vi "DCA Convert 1.5 to 1.8.vi"(1 "DCA 1.5 Test Parameters":T2={"Tag"="", "Use Instrument"=FALSE, "Quick Mode"=FALSE, "Topology"=enum."Pi", "Zo"=50.0, "Range"=0, "Resolution"=0, "Blank Screen"=FALSE, "Limits"=[], "Reports"={"Reports to Generate"=[], "Print Reports"=TRUE}, "Lock Topology"=FALSE, "Normalize"=TRUE, "ATTN Calc"=enum."Power"} {"Resolution" items=["Auto", "4 1/2", "5 1/2", "6 1/2"]; "Range" items=["Auto", "Min", "Max", "100", "1,000", "10,000", "100,000", "1,000,000", "10,000,000", "100,000,000"]}) -> (0 "DCA 1.8 Test Parameters":T1={"Tag"="", "Use Instrument"=FALSE, "Quick Mode"=FALSE, "Topology"=enum."Pi", "Zo"=50.0, "Range"=0, "Resolution"=0, "Blank Screen"=FALSE, "Limits"=[], "Datasheets"={"Datasheets to Generate"=[], "Print Datasheets"=TRUE}, "Lock Topology"=FALSE, "Normalize"=TRUE, "ATTN Calc"=enum."Power"} {"Resolution" items=["Auto", "4 1/2", "5 1/2", "6 1/2"]; "Range" items=["Auto", "Min", "Max", "100", "1,000", "10,000", "100,000", "1,000,000", "10,000,000", "100,000,000"]; "Limits"."Run" min=1 step=1})   [LabVIEW 2011]
uses:
  TypeDefs/DCA Test Parameters v1.5.ctl
  TypeDefs/DCA Test Parameters v1.8.ctl
panel:
  # "="
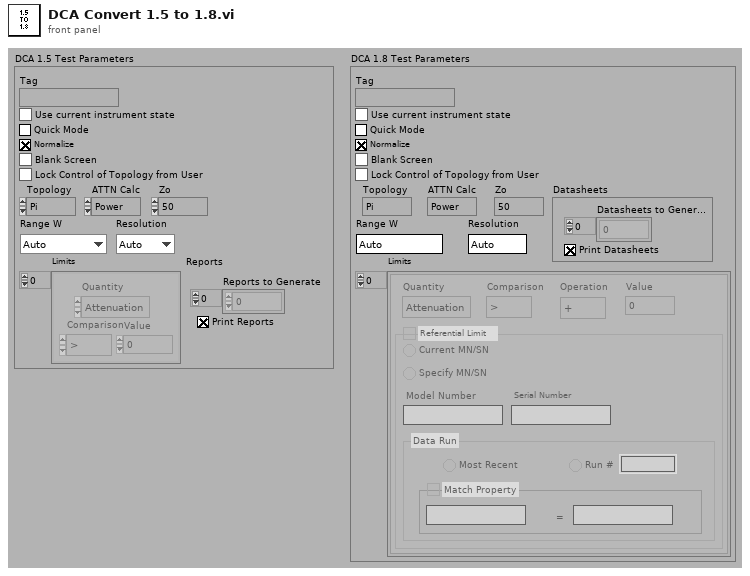
[diagram p1: front panel]
types:
  T1 = typedef "DCA Test Parameters v1.8.ctl" = cluster{"Tag":string, "Use Instrument":bool, "Quick Mode":bool, "Topology":enum32{"Pi", "T"}, "Zo":dbl, "Range":u16, "Resolution":u16, "Blank Screen":bool, "Limits":cluster{"Quantity":enum16{"Attenuation", "Zin", "Zout", "R1", "R2", "R3", "Rab", "Rac", "Rbc"}, "Comparison":enum16{">", ">=", "<", "<=", "+", "-"}, "Operation":enum16{"+", "-"}, "Value":dbl, "Ref Limit":bool, "Ref Type":enum32{"Current", "Specify"}, "Model":string, "Serial":string, "Run Type":enum32{"Most Recent", "Run #"}, "Run":i32, "Match Property":bool, "Property":string, "Property Value":string}[], "Datasheets":cluster{"Datasheets to Generate":i32[], "Print Datasheets":bool}, "Lock Topology":bool, "Normalize":bool, "ATTN Calc":enum32{"Power", "Voltage"}}
  T2 = typedef "DCA Test Parameters v1.5.ctl" = cluster{"Tag":string, "Use Instrument":bool, "Quick Mode":bool, "Topology":enum32{"Pi", "T"}, "Zo":dbl, "Range":u16, "Resolution":u16, "Blank Screen":bool, "Limits":cluster{"Quantity":enum16{"Attenuation", "Zin", "Zout", "R1", "R2", "R3", "Rab", "Rac", "Rbc"}, "Comparison":enum16{">", ">=", "<", "<=", "+", "-"}, "Value":dbl}[], "Reports":cluster{"Reports to Generate":i32[], "Print Reports":bool}, "Lock Topology":bool, "Normalize":bool, "ATTN Calc":enum32{"Power", "Voltage"}}
  T3 = cluster{"Quantity":enum16{"Attenuation", "Zin", "Zout", "R1", "R2", "R3", "Rab", "Rac", "Rbc"}, "Comparison":enum16{">", ">=", "<", "<=", "+", "-"}, "Operation":enum16{"+", "-"}, "Value":dbl, "Ref Limit":bool, "Ref Type":enum32{"Current", "Specify"}, "Model":string, "Serial":string, "Run Type":enum32{"Most Recent", "Run #"}, "Run":i32, "Match Property":bool, "Property":string, "Property Value":string}[]
  T4 = cluster{"Reports to Generate":i32[], "Print Reports":bool}
  T5 = cluster{"Quantity":enum16{"Attenuation", "Zin", "Zout", "R1", "R2", "R3", "Rab", "Rac", "Rbc"}, "Comparison":enum16{">", ">=", "<", "<=", "+", "-"}, "Value":dbl}[]
  T6 = cluster{"Quantity":enum16{"Attenuation", "Zin", "Zout", "R1", "R2", "R3", "Rab", "Rac", "Rbc"}, "Comparison":enum16{">", ">=", "<", "<=", "+", "-"}, "Operation":enum16{"+", "-"}, "Value":dbl, "Ref Limit":bool, "Ref Type":enum32{"Current", "Specify"}, "Model":string, "Serial":string, "Run Type":enum32{"Most Recent", "Run #"}, "Run":i32, "Match Property":bool, "Property":string, "Property Value":string}
  T7 = enum16{"Attenuation", "Zin", "Zout", "R1", "R2", "R3", "Rab", "Rac", "Rbc"}
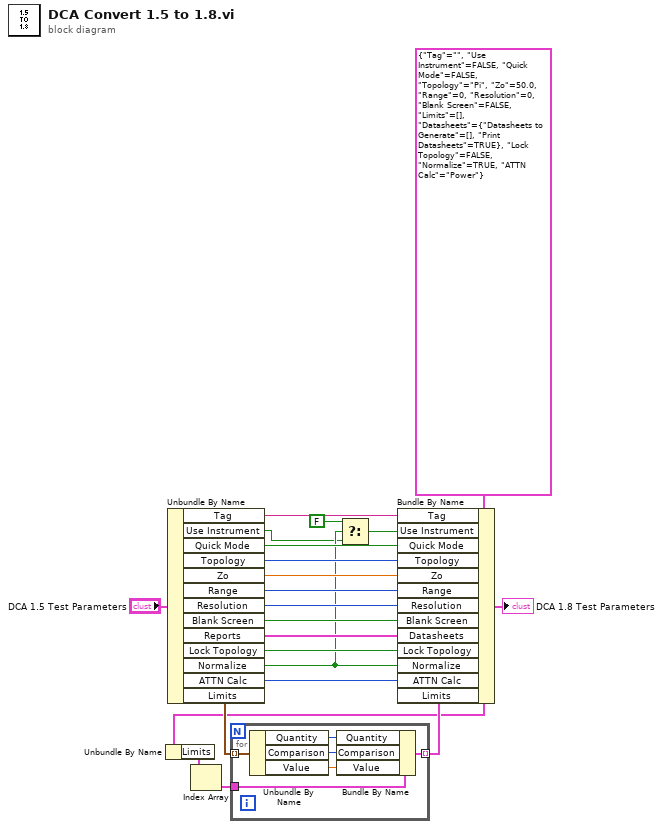
[diagram p0: block diagram]
diagram:
  w1 = T1 {"Tag"="", "Use Instrument"=FALSE, "Quick Mode"=FALSE, "Topology"=enum."Pi", "Zo"=50.0, "Range"=0, "Resolution"=0, "Blank Screen"=FALSE, "Limits"=[], "Datasheets"={"Datasheets to Generate"=[], "Print Datasheets"=TRUE}, "Lock Topology"=FALSE, "Normalize"=TRUE, "ATTN Calc"=enum."Power"} ("DCA 1.9 Test Parameters")
  n1 = Unbundle By Name(w1) -> ("Limits"=w12:T3)
  n2 = Unbundle By Name("DCA 1.5 Test Parameters") -> ("Tag"=w21:string, "Use Instrument"=w7:bool, "Quick Mode"=w20:bool, "Topology"=w19:enum32{"Pi", "T"}, "Zo"=w18:dbl, "Range"=w17:u16, "Resolution"=w16:u16, "Blank Screen"=w15:bool, "Reports"=w13:T4, "Lock Topology"=w14:bool, "Normalize"=w10:bool, "ATTN Calc"=w4:enum32{"Power", "Voltage"}, "Limits"=w5:T5)
  n3 = Index Array(array=w12) -> (element=w11:T6)  [unwired: 1 in]
  n4 = for {
    tunnel: w5 -> [w27] mode=indexing
    tunnel: w11 -> [w26]
    tunnel: [w22] -> w6 mode=indexing
    n5 = Unbundle By Name(w27) -> ("Quantity"=w23:T7, "Comparison"=w24:enum16{">", ">=", "<", "<=", "+", "-"}, "Value"=w25:dbl)
    n6 = Bundle By Name(cluster=w26, "Quantity"=w23, "Comparison"=w24, "Value"=w25) -> (w22:T6)
  }
  n7 = Select(t=FALSE, s=w10, f=w7) -> (s? t:f=w9:bool)
  n8 = Bundle By Name(cluster=w1, "Tag"=w21, "Use Instrument"=w9, "Quick Mode"=w20, "Topology"=w19, "Zo"=w18, "Range"=w17, "Resolution"=w16, "Blank Screen"=w15, "Datasheets"=w13, "Lock Topology"=w14, "Normalize"=w10, "ATTN Calc"=w4, "Limits"=w6) -> (→"DCA 1.8 Test Parameters":T1)
